vi "network.vi"() -> ()   [LabVIEW 2015]
uses:
  ctl/state.ctl
  keysight/keysight.lvclass
  R&S/RS.lvclass
  Database_util/Ctl/DNS.ctl
  Database_util/Ctl/database_Method.ctl
  network_Global/Global.vi
  network/network.lvclass
panel:
  in  "单通道测试":bool
  in  "测试":bool
  in  "网分校准":bool
  in  "connect":bool
  in  "Remote Address":refnum<visa-resource-name>="TCPIP0::192.168.1.253::inst0::INSTR"
  in  "Points":i32=101 caption="测量点数"
  in  "IF_Band":dbl=10.0 format="%.3f"
  in  "Stop":dbl=3900.0 format="%.3f"
  in  "Start":dbl=600.0 format="%.3f"
  in  "网分tab":enum32{"Keysight", "R&S"}(tab)
  in  "stop":bool
  in  "Limit":dbl=1.0
  in  "out":i32=4
  in  "in":i32=128
  out "消息":string
  # "dB"
  # "MHz"
  # "MHz"
  # "Point"
  # "kHz"
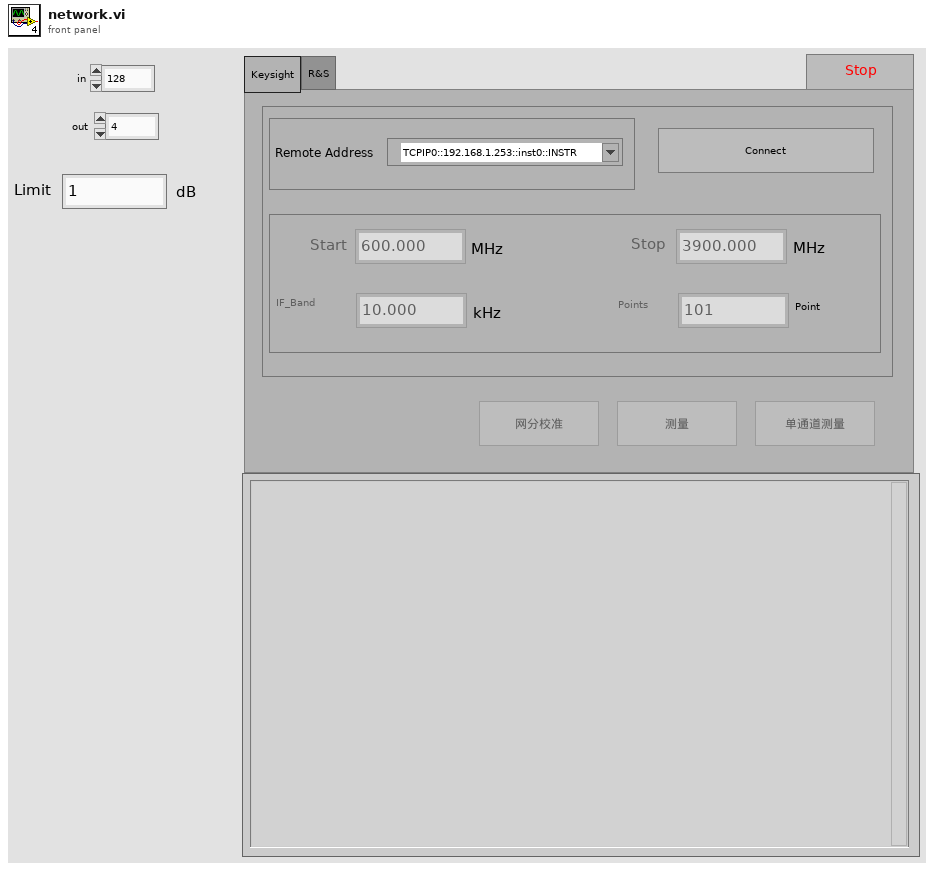
[diagram p1: front panel]
types:
  T1 = typedef "state.ctl" = enum16{"Idle", "直通基准测试", "校准基准测试", "校准直接测试", "导出基准数据", "导出差值数据"}
  T2 = typedef "database_Method.ctl" = enum16{"初始化", "查询", "关闭"}
  T3 = typedef "DNS.ctl" = string
  T4 = enum16{"Left Button", "Center Button", "Right Button", "Window Close"}
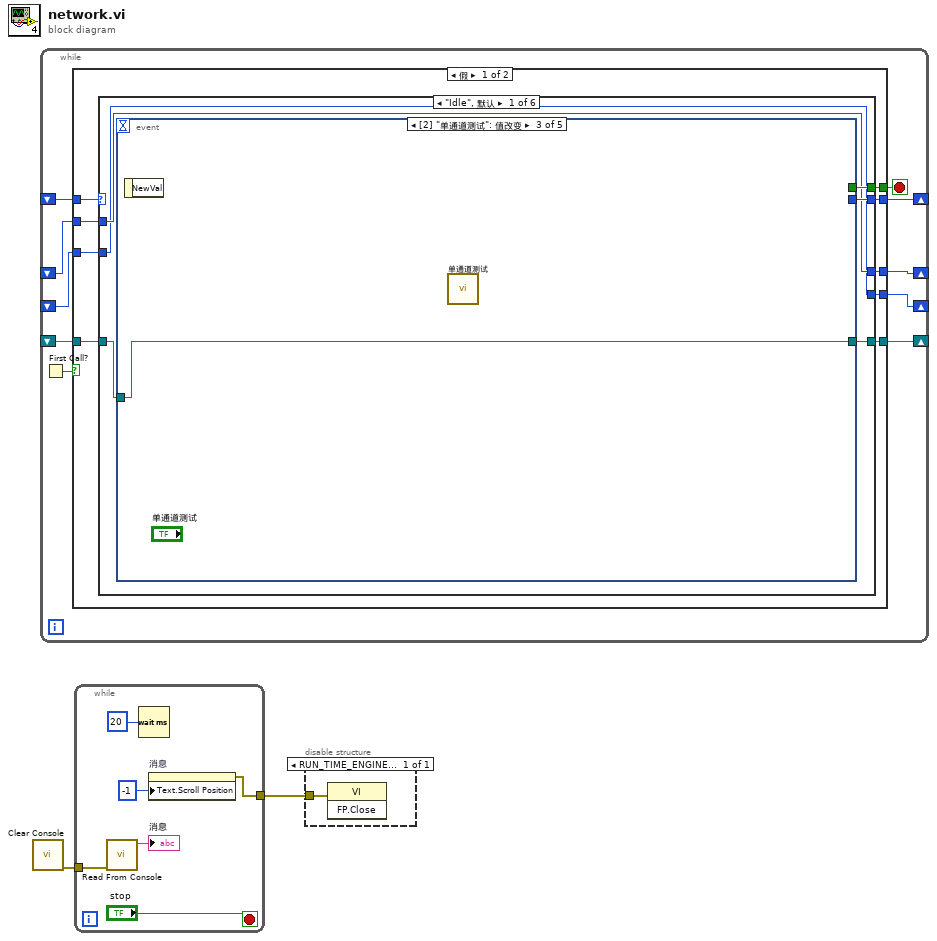
[diagram p0: block diagram]
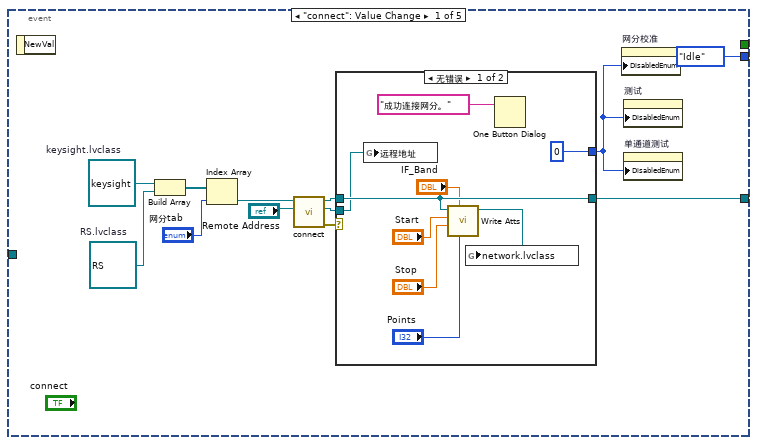
[diagram p2: hidden frame]
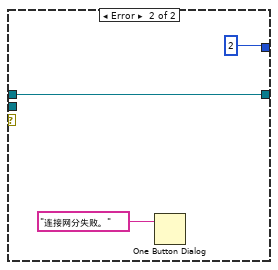
[diagram p3: hidden frame]
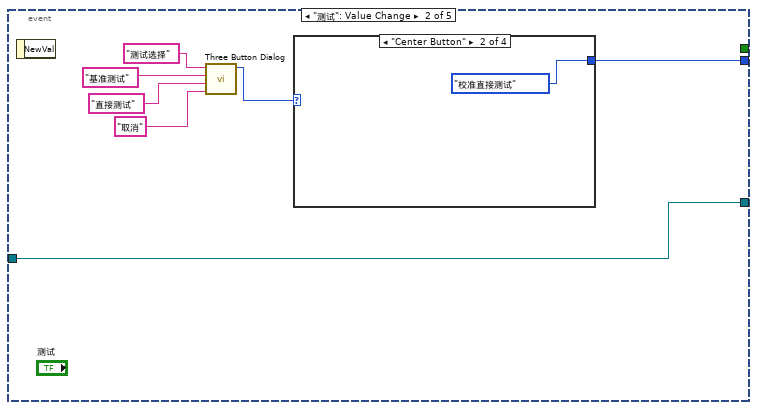
[diagram p4: hidden frame]
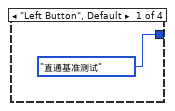
[diagram p5: hidden frame]
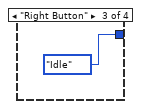
[diagram p6: hidden frame]
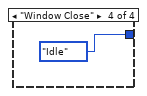
[diagram p7: hidden frame]
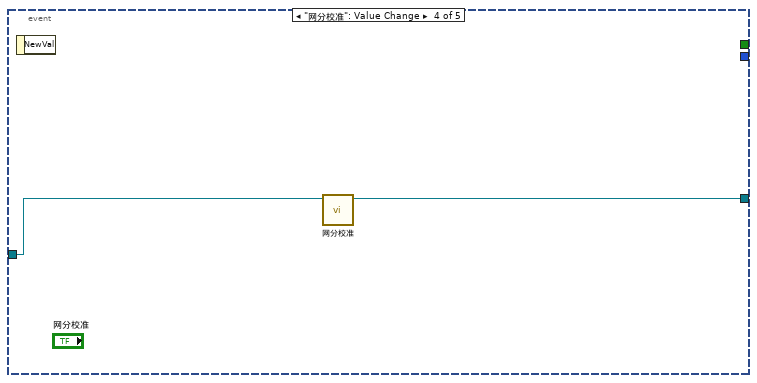
[diagram p8: hidden frame]
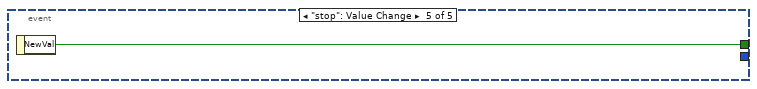
[diagram p9: hidden frame]
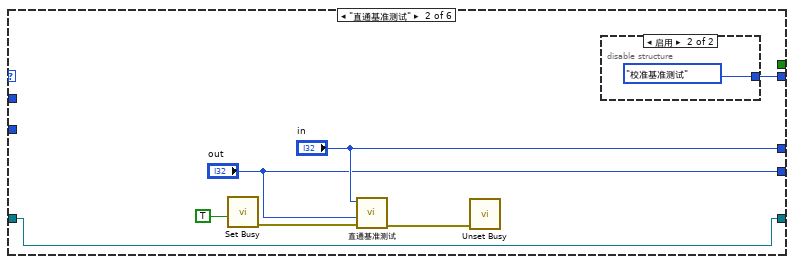
[diagram p10: hidden frame]
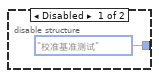
[diagram p11: hidden frame]
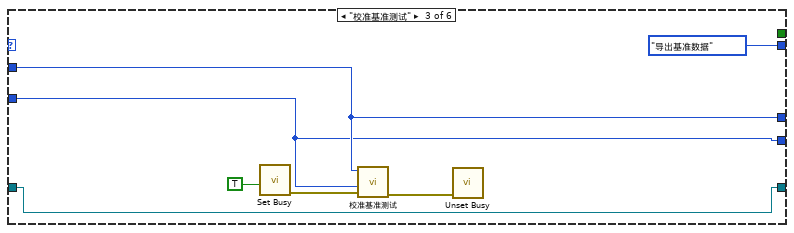
[diagram p12: hidden frame]
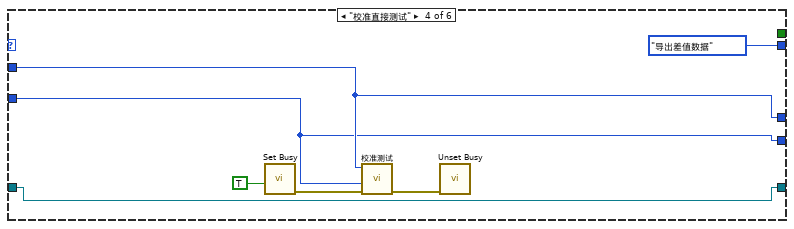
[diagram p13: hidden frame]
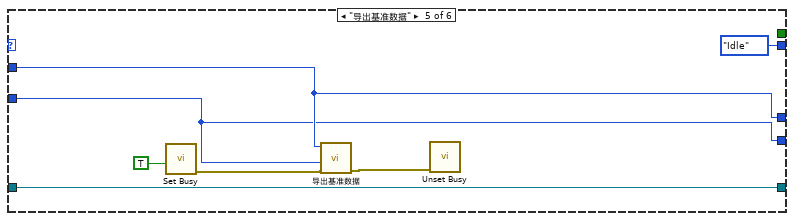
[diagram p14: hidden frame]
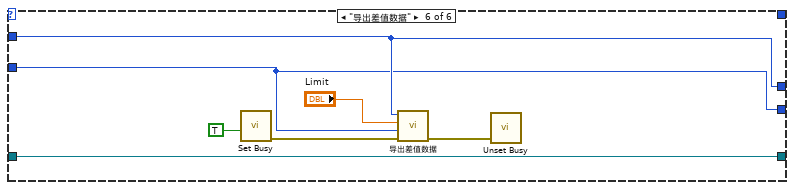
[diagram p15: hidden frame]
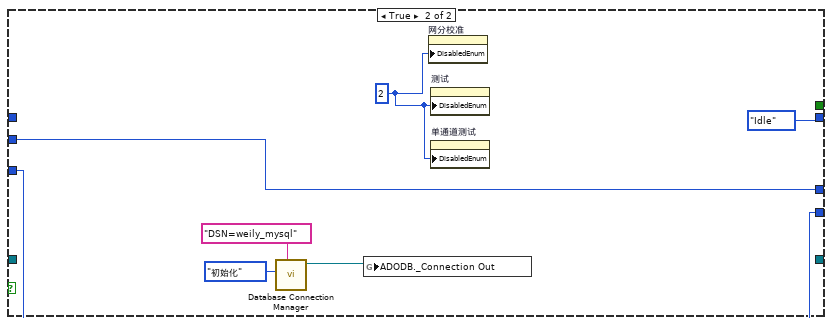
[diagram p16: hidden frame]
diagram:
  n1 = call "Clear Console.vi"() -> ("error out"=w2:errorcluster)  [unwired: 11 in]
  n2 = while {
    shift-right: [w10] -> _
    shift-left: _ -> [w11]
    shift-right: [w9] -> _
    shift-left: _ -> [w7]
    shift-right: [w6] -> _
    shift-left: _ -> [w4]
    shift-right: [w5] -> _
    shift-left: _ -> [w3]
    stop <- w12 stop-if-true
    n3 = First Call?() -> (First Call?: T/F=w8:bool)
    n4 = case shown="假" w8 {
      tunnel: [w21 _] -> w12
      tunnel: w11 -> [w20 _]
      tunnel: [w19 state."Idle" ("Enum")] -> w10
      tunnel: [w18 _] -> w9
      tunnel: w7 -> [w17 _]
      tunnel: w4 -> [w16 w109]
      tunnel: w3 -> [w15 w108]
      tunnel: [w14 w109] -> w6
      tunnel: [w13 w108] -> w5
      frame False {
        n5 = case shown="\"Idle\", 默认" w20 {
          tunnel: [w27 _ _ _ _ _] -> w21
          tunnel: [w26 w73 state."导出基准数据" ("Enum") state."导出差值数据" ("Enum") state."Idle" ("Enum") _] -> w19
          tunnel: [w25 w69 w78 w85 w92 w99] -> w18
          tunnel: w17 -> [w24 w69 w78 w85 w92 w99]
          tunnel: w16 -> [w23 _ w77 w84 w91 w98]
          tunnel: w15 -> [w22 _ w76 w83 w90 w97]
          tunnel: [w23 "in" w77 w84 w91 w98] -> w14
          tunnel: [w22 "out" w76 w83 w90 w97] -> w13
          frame "Idle", Default {
            n6 = event shown="[2] \"单通道测试\": 值改变" {
              selector: _ -> [_ _ _ _ _]
              dyn-events: _ -> [_ _ _ _ _]
              timeout: _ -> [_ _ _ _ _]
              tunnel: [_ _ _ _ w66] -> w27
              tunnel: [state."Idle" ("Enum") w53 _ _ _] -> w26
              tunnel: [w29 w52 w63 w64 _] -> w25
              tunnel: w24 -> [_ w52 w63 w65 _]
              event "connect": Value Change {
                w33 = refnum<class "RS.lvclass"> refnum  # RS.lvclass
                w32 = refnum<class "keysight.lvclass"> refnum  # keysight.lvclass
                n7 = event-data() -> ()  [unwired: 1 in, 1 out]
                n8 = Build Array(w32, w33) -> (w31:refnum<class "network.lvclass">[])
                n9 = Index Array(array=w31, index="网分tab") -> (element=w38:refnum<class "network.lvclass">)
                n10 = call-dynamic "connect.vi"("VISA resource name"="Remote Address", "network in"=w38) -> ("error out"=w37:errorcluster, "VISA resource name out"=w34:refnum<visa-resource-name>, "network out"=w30:refnum<class "network.lvclass">)  [unwired: 7 in]
                n11 = case shown="无错误" w37 {
                  tunnel: w34 -> [w42 _]
                  tunnel: w30 -> [w45 w50]
                  tunnel: [w45 w50] -> w29
                  tunnel: [0 2] -> w28
                  frame No Error {
                    n12 = global write "Global.vi" "远程地址"(w42) -> ()
                    n13 = call-dynamic "Write Atts.vi"("Points"="Points", "IF_Band"="IF_Band", "Stop"="Stop", "Start"="Start", "network in"=w45) -> ("network out"=w41:refnum<class "network.lvclass">)  [unwired: 5 in, 1 out]
                    n14 = global write "Global.vi" "network.lvclass"(w41) -> ()
                    n15 = One Button Dialog(message="成功连接网分。") -> ()  [unwired: 1 in, 1 out]
                  }
                  frame Error {
                    n16 = One Button Dialog(message="连接网分失败。") -> ()  [unwired: 1 in, 1 out]
                  }
                }
                n17 = property on="网分校准" class="Bool (严格)"("DisabledEnum"=w28) -> ()  [unwired: 2 in, 2 out]
                n18 = property on="测试" class="Bool (严格)"("DisabledEnum"=w28) -> ()  [unwired: 2 in, 2 out]
                n19 = property on="单通道测试" class="Bool (严格)"("DisabledEnum"=w28) -> ()  [unwired: 2 in, 2 out]
              }
              event "测试": Value Change {
                n20 = event-data() -> ()  [unwired: 1 in, 1 out]
                n21 = call <vilib>:"Three Button Dialog.vi"("Right Button Text (\"Cancel\")"="取消" ("Right Button Text (\"Cancel\")"), "Center Button Text (\"No\")"="直接测试" ("message"), "Left Button Text (\"Yes\")"="基准测试" ("message"), "message"="测试选择") -> ("Which Button?"=w54:T4)  [unwired: 7 in]
                n22 = case shown="\"Center Button\"" w54 {
                  tunnel: [state."直通基准测试" ("Enum") state."校准直接测试" ("Enum") state."Idle" ("Enum") state."Idle" ("Enum")] -> w53
                  frame "Left Button", Default {
                  }
                  frame "Center Button" {
                  }
                  frame "Right Button" {
                  }
                  frame "Window Close" {
                  }
                }
              }
              event "单通道测试": Value Change {
                n23 = event-data() -> ()  [unwired: 1 in, 1 out]
                n24 = call "单通道测试.vi"() -> ()  [unwired: 20 in]
              }
              event "网分校准": Value Change {
                n25 = event-data() -> ()  [unwired: 1 in, 1 out]
                n26 = call-dynamic "网分校准.vi"("network in"=w65) -> ("network out"=w64:refnum<class "network.lvclass">)  [unwired: 9 in, 1 out]
              }
              event "stop": Value Change {
                n27 = event-data() -> ("NewVal"=w66:bool)  [unwired: 1 in]
              }
            }
          }
          frame "直通基准测试" {
            n28 = call <vilib>:"Set Busy.vi"("disable click? (T)"=TRUE) -> ("error out"=w71:errorcluster)  [unwired: 9 in, 1 out]
            n29 = call "直通基准测试.vi"("error in (no error)"=w71, "out"="out", "in"="in") -> ("error out"=w70:errorcluster)  [unwired: 8 in]
            n30 = call <vilib>:"Unset Busy.vi"("error in (no error)"=w70) -> ()  [unwired: 10 in, 1 out]
            n31 = disable-structure shown="启用" {
              disable-tunnel: [state."校准基准测试" ("Enum") state."校准基准测试" ("Enum")] -> w73
              frame Disabled {
              }
              frame Enabled {
              }
            }
          }
          frame "校准基准测试" {
            n32 = call <vilib>:"Set Busy.vi"("disable click? (T)"=TRUE) -> ("error out"=w81:errorcluster)  [unwired: 9 in, 1 out]
            n33 = call "校准基准测试.vi"("error in (no error)"=w81, "out"=w76, "in"=w77) -> ("error out"=w80:errorcluster)  [unwired: 8 in]
            n34 = call <vilib>:"Unset Busy.vi"("error in (no error)"=w80) -> ()  [unwired: 10 in, 1 out]
          }
          frame "校准直接测试" {
            n35 = call <vilib>:"Set Busy.vi"("disable click? (T)"=TRUE) -> ("error out"=w87:errorcluster)  [unwired: 9 in, 1 out]
            n36 = call "校准测试.vi"("error in (no error)"=w87, "out"=w83, "in"=w84) -> ("error out"=w86:errorcluster)  [unwired: 8 in]
            n37 = call <vilib>:"Unset Busy.vi"("error in (no error)"=w86) -> ()  [unwired: 10 in, 1 out]
          }
          frame "导出基准数据" {
            n38 = call <vilib>:"Set Busy.vi"("disable click? (T)"=TRUE) -> ("error out"=w94:errorcluster)  [unwired: 9 in, 1 out]
            n39 = call "导出基准数据.vi"("error in"=w94, "OUT"=w90, "IN"=w91) -> ("error out"=w93:errorcluster)  [unwired: 8 in]
            n40 = call <vilib>:"Unset Busy.vi"("error in (no error)"=w93) -> ()  [unwired: 10 in, 1 out]
          }
          frame "导出差值数据" {
            n41 = call <vilib>:"Set Busy.vi"("disable click? (T)"=TRUE) -> ("error out"=w101:errorcluster)  [unwired: 9 in, 1 out]
            n42 = call "导出差值数据.vi"("error in"=w101, "COM"=w97, "阀值"="Limit", "IN"=w98) -> ("error out"=w102:errorcluster)  [unwired: 7 in]
            n43 = call <vilib>:"Unset Busy.vi"("error in (no error)"=w102) -> ()  [unwired: 10 in, 1 out]
          }
        }
      }
      frame True {
        w107 = 2
        n44 = call "Database Connection Manager.vi"("ConnectionString"=T3 "DSN=weily_mysql", "Method"=database_Method."初始化") -> ("ADODB._Connection Out"=w104:refnum<k7>)  [unwired: 6 in, 3 out]
        n45 = global write "Global.vi" "ADODB._Connection Out"(w104) -> ()
        n46 = property on="网分校准" class="Bool (严格)"("DisabledEnum"=w107) -> ()  [unwired: 2 in, 2 out]
        n47 = property on="测试" class="Bool (严格)"("DisabledEnum"=w107) -> ()  [unwired: 2 in, 2 out]
        n48 = property on="单通道测试" class="Bool (严格)"("DisabledEnum"=w107) -> ()  [unwired: 2 in, 2 out]
      }
    }
  }
  n49 = while {
    tunnel: w2 -> [w115]
    tunnel: [w111] -> w1
    stop <- "stop" stop-if-true
    n50 = call "Read From Console.vi"("error in (no error)"=w115) -> ("Output"=→"消息":string)  [unwired: 9 in, 1 out]
    n51 = Wait (ms)(milliseconds to wait=u32 20) -> ()  [unwired: 1 out]
    n52 = property on="消息" class="Str"("Text.Scroll Position"=i8 -1 ("milliseconds to wait")) -> (error out=w111:errorcluster)  [unwired: 2 in, 1 out]
  }
  n53 = disable-structure shown="RUN_TIME_ENGINE==True, default" {
    disable-tunnel: w1 -> [w117]
    frame condition #0 (active) {
      n54 = invoke class="VI" method="FP.Close"(error in=w117) -> ()  [unwired: 2 in, 3 out]
    }
  }
